vi "macro_LinearSystemLoop_DiffDrv_ID_Execute.vi"() -> ()   [LabVIEW 2019, in "Trajectory_Library.lvlib"]
uses:
  Trajectory_Library.lvlib
  LinearSystemId_IdentifyDriveTrainSystem.vi
  LinearSystem_New.vi
  MatBuilder_Create.vi
  MatrixHelper_Zero.vi
  MatBuilder_Fill.vi
  MatrixHelper_CoerceSize.vi
panel:
  out "Left Motor Dmd":dbl
  out "Right Motor Dmd":dbl
  in  "Left Vel SP m/s":dbl
  in  "Right Vel SP m/s":dbl
  in  "Left Vel PV m/s":dbl
  in  "Right Vel PV m/s":dbl
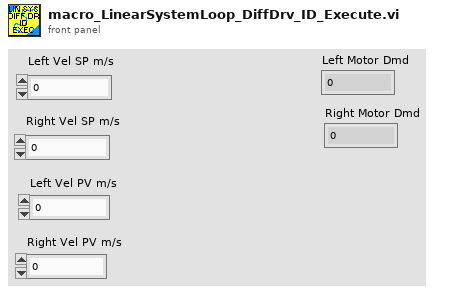
[diagram p1: front panel]
types:
  T1 = typedef "Trajectory_Library.lvlib/LINEAR_SYSTEM_LOOP_DIFF_DRV_CTRL_PARAMS.CTL" = cluster{"Left Vel Model Std Dev m/s":dbl, "Left Vel Meas Std Dev m/s":dbl, "Left Vel Ctrl Tol m/s":dbl, "Max Control Effort":dbl, "Right Vel Ctrl Tol m/s":dbl, "Right Vel Meas Std Dev m/s":dbl, "Right Vel Model Std Dev m/s":dbl}
  T2 = typedef "Trajectory_Library.lvlib/LINEAR_SYSTEM.ctl" = cluster{"m_A":T3, "m_B":T3, "m_C":T3, "m_D":T3, "States":i32, "Inputs":i32, "Outputs":i32}
  T3 = typedef "NI_Matrix.lvlib/RealMatrix.ctl" = dbl[][]
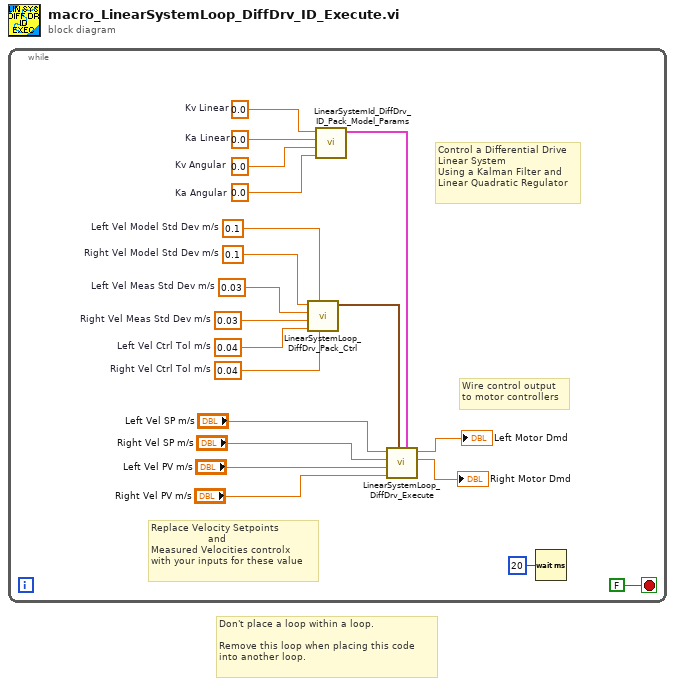
[diagram p0: block diagram]
diagram:
  # "Don't place a loop within a loop.\n \nRemove this loop when placing this code\ninto another loop."
  n1 = while {
    stop <- FALSE stop-if-true
    w1 = 0.0  # Kv Linear
    w2 = 0.0  # Ka Linear
    w3 = 0.0  # Kv Angular
    w4 = 0.0  # Ka Angular
    w12 = 0.1  # Right Vel Model Std Dev m/s
    w13 = 0.03  # Left Vel Meas Std Dev m/s
    w14 = 0.03  # Right Vel Meas Std Dev m/s
    w15 = 0.04  # Left Vel Ctrl Tol m/s
    w16 = 0.1  # Left Vel Model Std Dev m/s
    w17 = 0.04  # Right Vel Ctrl Tol m/s
    # "Wire control output\nto motor controllers"
    # "Replace Velocity Setpoints \n                   and \nMeasured Velocities controlx\nwith your inputs for these value"
    # "Control a Differential Drive\nLinear System\nUsing a Kalman Filter and \nLinear Quadratic Regulator"
    n2 = call "LinearSystemLoop_DiffDrv_Pack_Ctrl.vi"("Right Vel Ctrl Tol m/s"=w17, "Left Vel Model Std Dev m/s"=w16, "Left Vel Ctrl Tol m/s"=w15, "Right Vel Meas Std Dev m/s"=w14, "Left Vel Meas Std Dev m/s"=w13, "Right Vel Model Std Dev m/s"=w12) -> ("LinearSystemLoop_DiffDrv_Ctrl_Params"=w18:T1)  [unwired: 5 in]
    n3 = call "LinearSystemId_DiffDrv_ID_Pack_Model_Params.vi"("Ka Angular"=w4, "Kv Angular"=w3, "Ka Linear"=w2, "Kv Linear"=w1) -> ("DiffDrv_LinearSystem"=w5:T2)  [unwired: 7 in]
    n4 = call "LinearSystemLoop_DiffDrv_Execute.vi"("Linear System"=w5, "LinearSystemLoop_DiffDrv_Control_Params"=w18, "Right Vel PV m/s"="Right Vel PV m/s", "Left Vel PV m/s"="Left Vel PV m/s", "Right Vel SP m/s"="Right Vel SP m/s", "Left Vel SP m/s"="Left Vel SP m/s") -> ("Right Motor Dmd"=→"Right Motor Dmd":dbl, "Left Motor Dmd"=→"Left Motor Dmd":dbl)  [unwired: 1 in, 3 out]
    n5 = Wait (ms)(milliseconds to wait=u32 20) -> ()  [unwired: 1 out]
  }
